vi "EEI EXP8.vi"() -> ()   [LabVIEW 2020]
panel:
  out "String 2":string
  out "Boolean 4":bool
  out "Boolean 3":bool
  out "Numeric 2":dbl
  out "output cluster":T1
  in  "String":string
  in  "Boolean 2":bool
  in  "Numeric":dbl
  in  "Boolean":bool
  out "all lower case string":string
  out "all upper case string":string
  in  "string 7":string
  in  "string 6":string
  out "replaced substring":string
  out "result string":string
  in  "length (len. of substring)":i32
  in  "offset (0) 3":i32
  in  "substring (\"\")":string
  in  "string 5":string
  out "current time":timestamp
  out "substring":string
  in  "length (rest)":i32
  in  "offset (0)":i32
  in  "string 4":string
  out "concatenated string":string
  in  "string 3":string
  in  "string 2":string
  out "length":i32
  in  "string":string
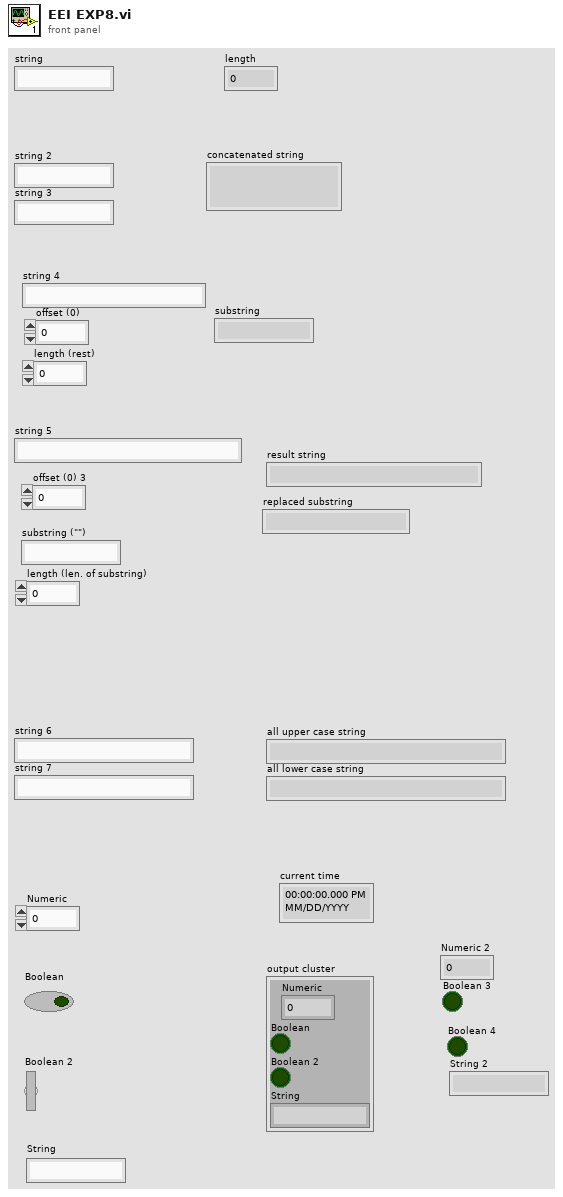
[diagram p1: front panel]
types:
  T1 = cluster{"Numeric":dbl, "Boolean":bool, "Boolean 2":bool, "String":string}
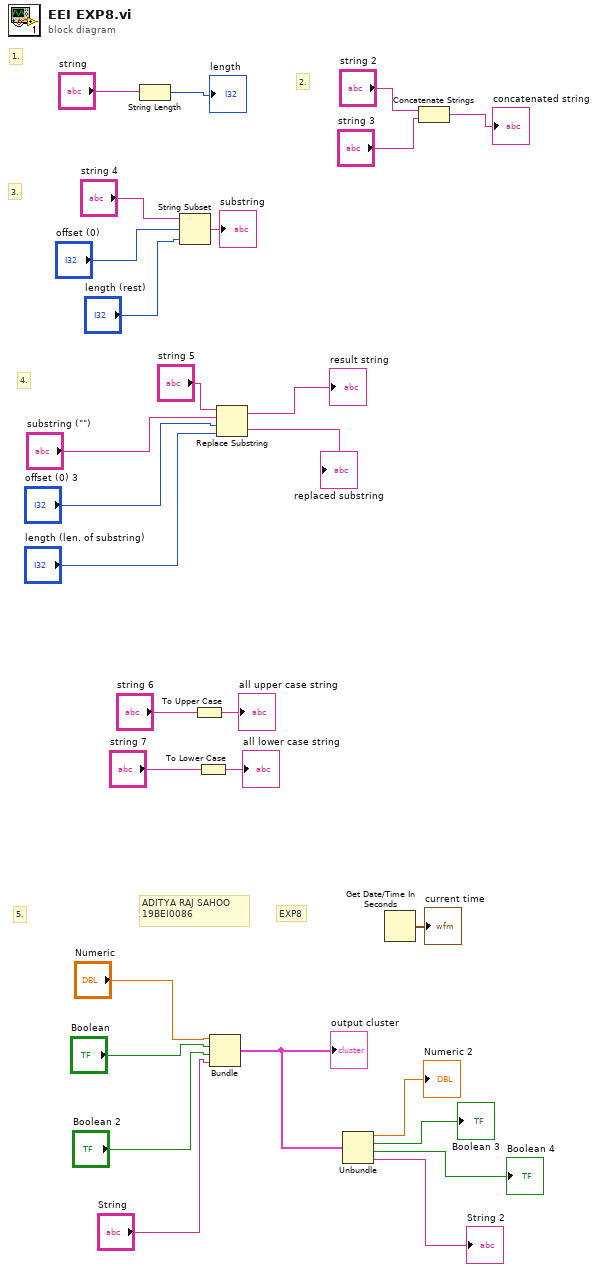
[diagram p0: block diagram]
diagram:
  # "5."
  # "EXP8"
  # "ADITYA RAJ SAHOO\n19BEI0086"
  # "4."
  # "3."
  # "2."
  # "1."
  n1 = String Length(string="string") -> (length=→"length":i32)
  n2 = String Subset(string="string 4", offset (0)="offset (0)", length (rest)="length (rest)") -> (substring=→"substring":string)
  n3 = To Upper Case(1:"string 6") -> (0:→"all upper case string":string)
  n4 = To Lower Case(string="string 7") -> (all lower case string=→"all lower case string":string)
  n5 = Bundle("Numeric"="Numeric", "Boolean"="Boolean", "Boolean 2"="Boolean 2", "String"="String") -> (w5:T1)  [unwired: 1 in]
  "output cluster" <- w5
  n6 = Replace Substring(2:"length (len. of substring)", 3:"offset (0) 3", 4:"substring (\"\")", 5:"string 5") -> (0:→"replaced substring":string, 1:→"result string":string)
  n7 = Unbundle(w5) -> ("Numeric"=→"Numeric 2":dbl, "Boolean"=→"Boolean 3":bool, "Boolean 2"=→"Boolean 4":bool, "String"=→"String 2":string)
  n8 = Get Date/Time In Seconds() -> (seconds since 1Jan1904=→"current time":timestamp)
  n9 = Concatenate Strings("string 2", "string 3") -> (→"concatenated string":string)
